vi "Illumination Tests_2.vi"(0 "Test Number":i32, 5 "FileName":path=path "c:/$safe$.bmp", 7 "Pixel Offset":i32, 9 "Pixel Average":i32) -> (1 "Hor Max":sgl format="%.2g", 2 "Vert Max":sgl format="%#.2g", 3 "Gray Level Intensity":T2 {"Standard  Deviation" format="%.2f"; "Mean Intensity" format="%.2f"; "Maximum Intensity" format="%.2f"; "Minimum Intensity" format="%.2f"}, 4 "Mean Intensity":sgl, 6 "Horz Ratio":sgl format="%#.2g", 10 "Vert Ratio":sgl format="%#.2g", 12 "Horz Min":sgl format="%.2g", 14 "Vert Min":sgl format="%#.2g", 15 "error out":errorcluster)   [LabVIEW 2014]
uses:
  <vilib>/vision/NI_Vision_Development_Module.lvlib
panel:
  out "Y Resolution":i32
  out "X Resolution":i32
  out "Image":T1(plugin-control)
  out "Vertical Averages":sgl[](array[numeric]) format="%#.2g"
  out "Horizontal Averages":sgl[](array[numeric]) format="%#.2g"
  in  "error in (no error)":errorcluster
  # "0 = Center Illumination Brightness\n1 = Uniformity\n2 = Spot Color Test"
  # "UNIFORMITY"
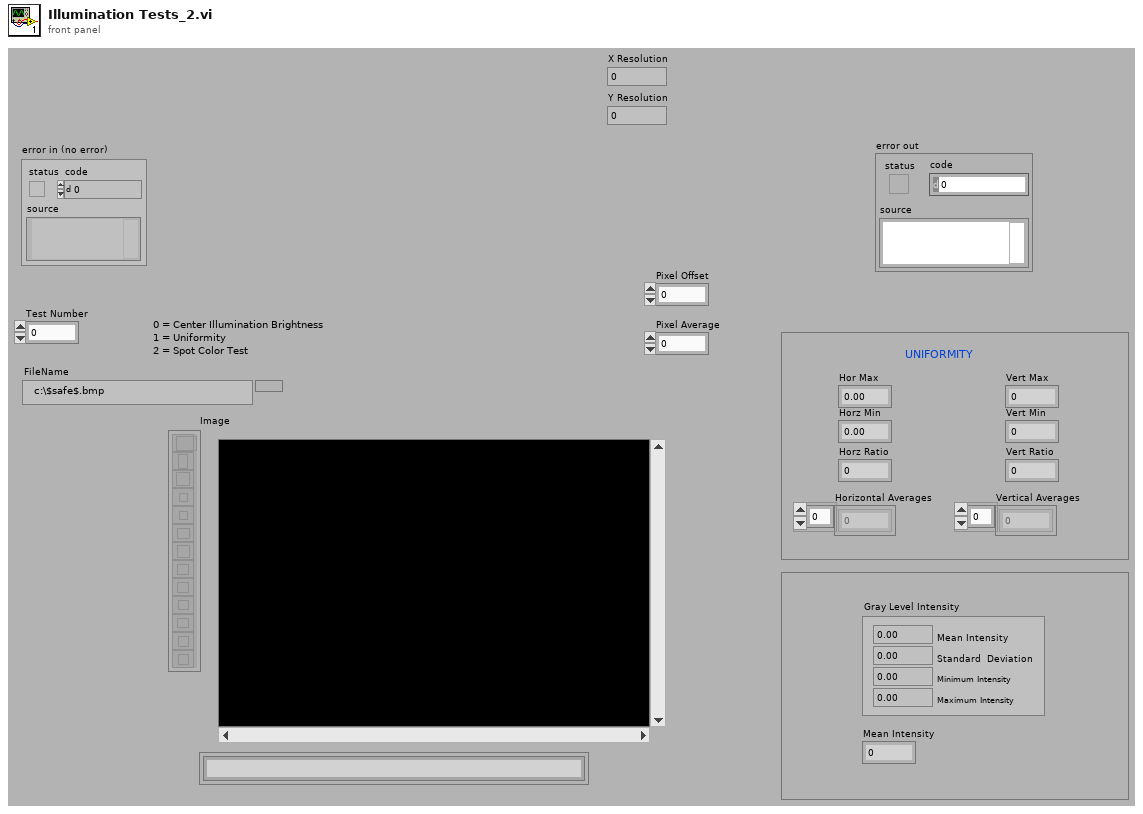
[diagram p1: front panel]
types:
  T1 = typedef "IMAQ Image.ctl" = refnum<image>
  T2 = cluster{"Mean Intensity":sgl, "Standard  Deviation":sgl, "Minimum Intensity":sgl, "Maximum Intensity":sgl}
  T3 = typedef "IMAQ Rectangle" = cluster{"Left":i32, "Top":i32, "Right":i32, "Bottom":i32, "Rotation":dbl}
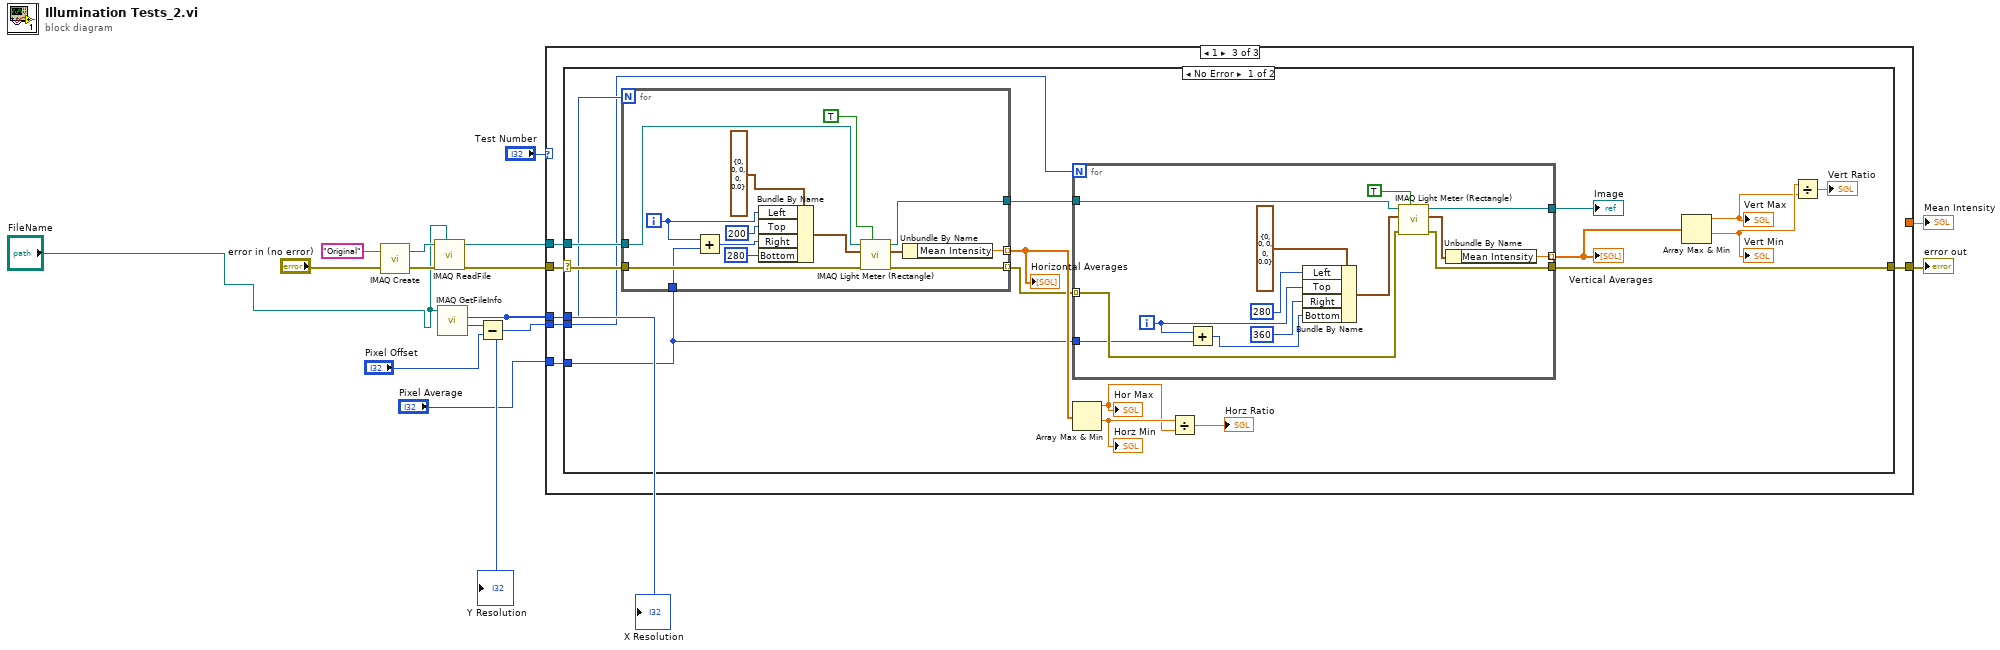
[diagram p0: block diagram]
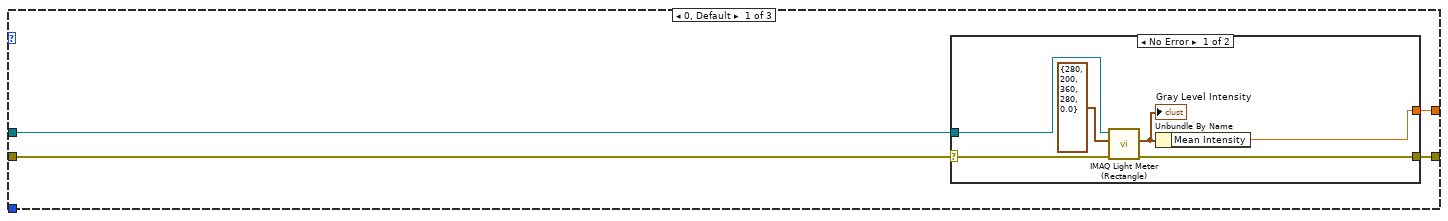
[diagram p2: hidden frame]
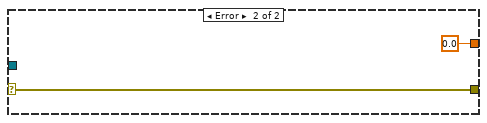
[diagram p3: hidden frame]
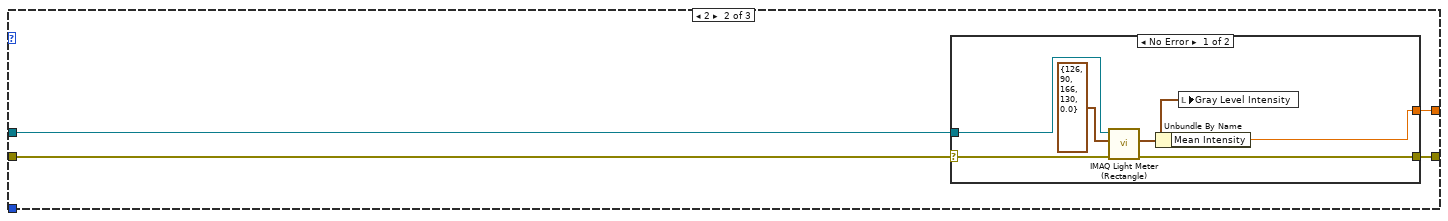
[diagram p4: hidden frame]
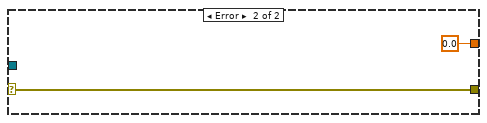
[diagram p5: hidden frame]
diagram:
  n1 = call "IMAQ Create"("Image Name"="Original", "error in (no error)"="error in (no error)") -> ("New Image"=w14:T1, "error out"=w11:errorcluster)  [unwired: 3 in]
  n2 = call "IMAQ ReadFile"("File Path"="FileName", "error in (no error)"=w11, "Image"=w14) -> ("error out"=w10:errorcluster, "Image Out"=w13:T1)  [unwired: 4 in, 3 out]
  n3 = call "IMAQ GetFileInfo"("File Path"="FileName") -> ("Y Resolution"=w4:i32, "X Resolution"=w6:i32)  [unwired: 4 in, 5 out]
  "X Resolution" <- w6
  "Y Resolution" <- w4
  n4 = Subtract(x=w4, y="Pixel Offset") -> (x-y=w5:i32)
  n5 = case shown="1" "Test Number" {
    tunnel: w13 -> [w19 w31 w43]
    tunnel: w10 -> [w18 w30 w45]
    tunnel: [w17 w29 _] -> w9
    tunnel: [w16 w28 w44] -> w8
    tunnel: w6 -> [_ _ w42]
    tunnel: w5 -> [_ _ w41]
    tunnel: "Pixel Average" -> [_ _ w40]
    frame 0, Default {
      n6 = case shown="No Error" w18 {
        selector: w18 -> [w20 w26]
        tunnel: w19 -> [w24 _]
        tunnel: [w22 sgl 0.0 ("Mean Intensity")] -> w17
        tunnel: [w21 w26] -> w16
        frame No Error {
          n7 = call "IMAQ Light Meter (Rectangle)"("error in (no error)"=w20, "Rectangle"=T3 {"Left"=280, "Top"=200, "Right"=360, "Bottom"=280, "Rotation"=0.0}, "Image"=w24) -> ("error out"=w21:errorcluster, "Gray Level Intensities"=w23:T2)  [unwired: 4 in, 3 out]
          "Gray Level Intensity" <- w23
          n8 = Unbundle By Name(w23) -> ("Mean Intensity"=w22:sgl)
        }
        frame Error {
        }
      }
    }
    frame 2 {
      n9 = case shown="No Error" w30 {
        selector: w30 -> [w33 w38]
        tunnel: w31 -> [w36 _]
        tunnel: [w35 sgl 0.0 ("Mean Intensity")] -> w29
        tunnel: [w34 w38] -> w28
        frame No Error {
          n10 = call "IMAQ Light Meter (Rectangle)"("error in (no error)"=w33, "Rectangle"=T3 {"Left"=126, "Top"=90, "Right"=166, "Bottom"=130, "Rotation"=0.0}, "Image"=w36) -> ("error out"=w34:errorcluster, "Gray Level Intensities"=w32:T2)  [unwired: 4 in, 3 out]
          n11 = Unbundle By Name(w32) -> ("Mean Intensity"=w35:sgl)
          n12 = local write "Gray Level Intensity"(w32) -> ()
        }
        frame Error {
        }
      }
    }
    frame 1 {
      n13 = case shown="No Error" w45 {
        selector: w45 -> [w53 w91]
        tunnel: [w52 w91] -> w44
        tunnel: w43 -> [w49 _]
        tunnel: w42 -> [w48 _]
        tunnel: w41 -> [w47 _]
        tunnel: w40 -> [w46 _]
        frame No Error {
          n14 = for {
            N: w48 -> [_]
            tunnel: [w83] -> w62 mode=indexing
            tunnel: w49 -> [w81]
            tunnel: [w80] -> w54 mode=indexing
            tunnel: w53 -> [w79]
            tunnel: [w78] -> w51
            tunnel: w46 -> [w77]
            i -> [w88]
            n15 = Add(x=w88, y=w77) -> (x+y=w87:i32)
            n16 = Bundle By Name(cluster=T3 {"Left"=0, "Top"=0, "Right"=0, "Bottom"=0, "Rotation"=0.0} ("Rectangle"), "Left"=w88, "Top"=200, "Right"=w87, "Bottom"=280) -> (w85:T3)
            n17 = call "IMAQ Light Meter (Rectangle)"("Show Search Area"=TRUE, "error in (no error)"=w79, "Rectangle"=w85, "Image"=w81) -> ("error out"=w80:errorcluster, "Gray Level Intensities"=w84:T2, "Image Out"=w78:T1)  [unwired: 3 in, 2 out]
            n18 = Unbundle By Name(w84) -> ("Mean Intensity"=w83:sgl)
          }
          "Horizontal Averages" <- w62
          n19 = for {
            N: w47 -> [_]
            tunnel: [w73] -> w61 mode=indexing
            tunnel: [w72] -> w52
            tunnel: w54 -> [w66] mode=indexing
            tunnel: w51 -> [w65]
            tunnel: [w64] -> w50
            tunnel: w46 -> [w63]
            i -> [w69]
            n20 = Add(x=w69, y=w63) -> (x+y=w67:i32)
            n21 = Bundle By Name(cluster=T3 {"Left"=0, "Top"=0, "Right"=0, "Bottom"=0, "Rotation"=0.0} ("Rectangle"), "Left"=280 ("Top"), "Top"=w69, "Right"=360 ("Bottom"), "Bottom"=w67) -> (w75:T3)
            n22 = call "IMAQ Light Meter (Rectangle)"("Show Search Area"=TRUE, "error in (no error)"=w66, "Rectangle"=w75, "Image"=w65) -> ("error out"=w72:errorcluster, "Gray Level Intensities"=w74:T2, "Image Out"=w64:T1)  [unwired: 3 in, 2 out]
            n23 = Unbundle By Name(w74) -> ("Mean Intensity"=w73:sgl)
          }
          "Vertical Averages" <- w61
          "Image" <- w50
          n24 = Array Max & Min(array=w62) -> (max value=w57:sgl, min value=w58:sgl)  [unwired: 2 out]
          "Hor Max" <- w57
          "Horz Min" <- w58
          n25 = Divide(x=w58, y=w57) -> (x/y=→"Horz Ratio":sgl)
          n26 = Array Max & Min(array=w61) -> (max value=w59:sgl, min value=w60:sgl)  [unwired: 2 out]
          "Vert Max" <- w59
          "Vert Min" <- w60
          n27 = Divide(x=w60, y=w59) -> (x/y=→"Vert Ratio":sgl)
        }
        frame Error {
        }
      }
    }
  }
  "Mean Intensity" <- w9
  "error out" <- w8
